vi "Wait for Run Button.vi"(6 "STOP refnum":refnum<vi>, 7 "RUN refnum":refnum<vi>, 8 "error in":errorcluster, 11 "status message (Running.)":string="Running.") -> (0 "error out":errorcluster, 2 "Run":bool)   [LabVIEW 2020]
doc: "This function performs the following:\n\n1) Enable the RUN button and Disable and Gray Out the STOP button.\n2) Wait for the RUN button to be pressed or error status is TRUE (error). \n (Poll at 50 ms interval, with no timeout.)\n3) If error status is FALSE (no error), then set the error cluster source string to \"Running\".\n (Error status will remain FALSE.)\n4) Enable the STOP button and Disable and Gray Out the RUN button.\n\nIf the input error status is TRUE (error), then no button attributes are changed, no polling occurs, and the existing error cluster is unchanged."
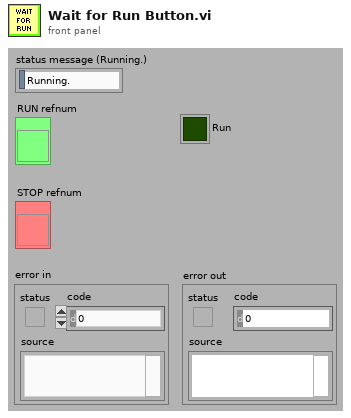
[diagram p1: front panel]
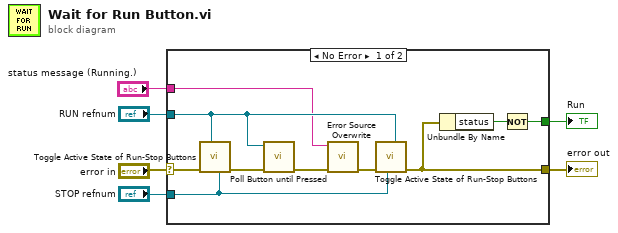
[diagram p0: block diagram]
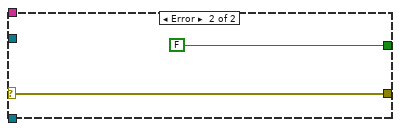
[diagram p2: hidden frame]
diagram:
  n1 = case shown="No Error" "error in" {
    selector: "error in" -> [w16 w18]
    tunnel: [w9 w18] -> w6
    tunnel: "RUN refnum" -> [w13 _]
    tunnel: "STOP refnum" -> [w15 _]
    tunnel: "status message (Running.)" -> [w10 _]
    tunnel: [w7 FALSE] -> w1
    frame No Error {
      n2 = call "Toggle Active State of Run-Stop Buttons.vi"("inactive button refnum"=w15, "active button refnum"=w13, "error in"=w16) -> ("error out"=w14:errorcluster)  [unwired: 6 in]
      n3 = call "Poll Button until Pressed.vi"("error in"=w14, "button refnum"=w13) -> ("error out"=w12:errorcluster)  [unwired: 6 in, 1 out]
      n4 = call "Error Source Overwrite.vi"("error in"=w12, "source"=w10) -> ("error out"=w11:errorcluster)  [unwired: 7 in]
      n5 = call "Toggle Active State of Run-Stop Buttons.vi"("inactive button refnum"=w13, "active button refnum"=w15, "error in"=w11) -> ("error out"=w9:errorcluster)  [unwired: 6 in]
      n6 = Unbundle By Name(w9) -> ("status"=w8:bool)
      n7 = Not(x=w8) -> (.not. x?=w7:bool)
    }
    frame Error {
    }
  }
  "error out" <- w6
  "Run" <- w1
